vi "StorageRefnumProbe.vi"(1 "dup storage refnum":refnum<k20>) -> (0 "stop":bool)   [LabVIEW 2017]
uses:
  <resource>/objmgr/Storage.rc
panel:
  in  "Invalid refnum":string="INVALID REFNUM"
  in  "Tab Control":T1(tab)
  in  "Storage parameters":i32(listbox)
  out "USI Storage type":string
  out "Object type:":string
  in  "Properties":i32(listbox)
  in  "Data values":i32(listbox)
  out "Waveform Graph":dynamicdata(graph)
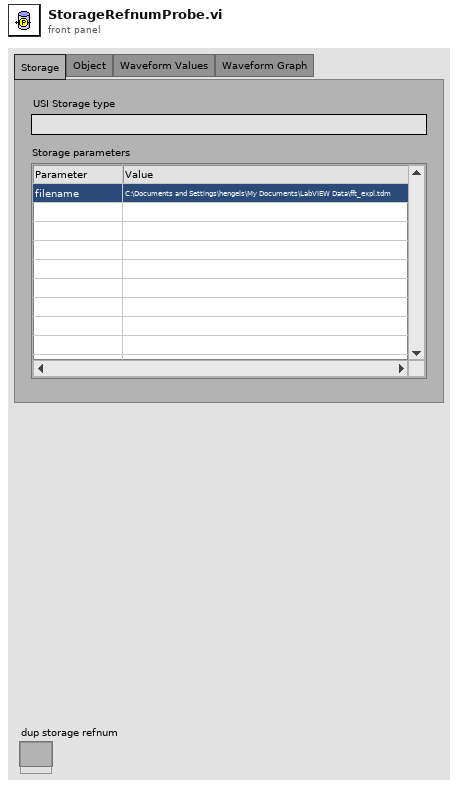
[diagram p1: front panel]
types:
  T1 = enum32{"Storage", "Object", "Waveform Values", "Waveform Graph"}
  T2 = enum32{"Page Enabled", "Page Disabled", "Page Disabled & Grayed"}
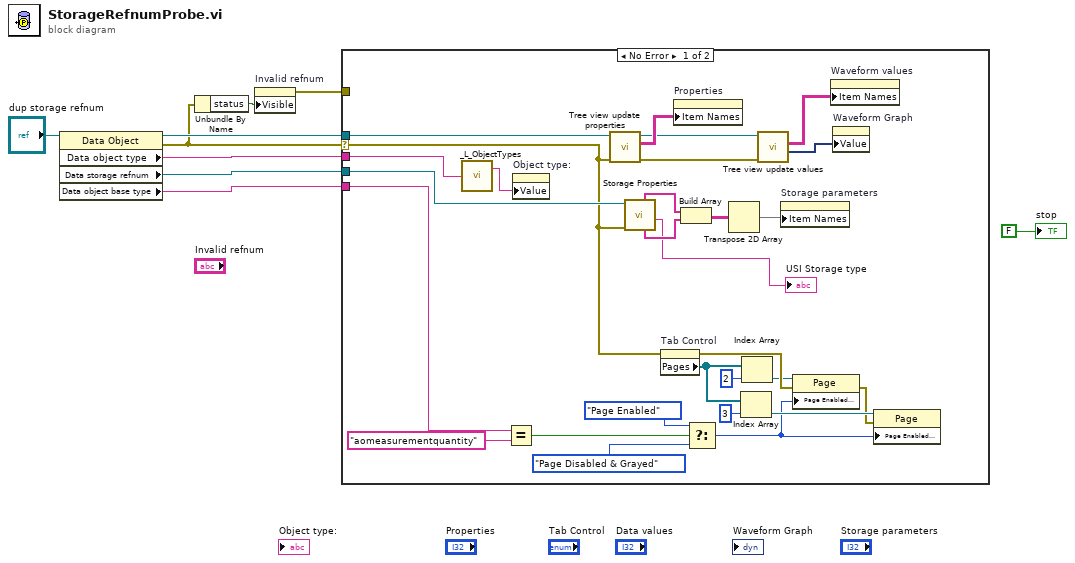
[diagram p0: block diagram]
diagram:
  n1 = property class="Data Object"(reference="dup storage refnum") -> (reference out=w9:refnum<k20>, error out=w3:errorcluster, "Data object type"=w5:string, "Data storage refnum"=w8:refnum<k20>, "Data object base type"=w7:string)  [unwired: 1 in]
  n2 = Unbundle By Name(w3) -> ("status"=w1:bool)
  n3 = property on="Invalid refnum" class="Str"("Visible"=w1) -> (error out=w2:errorcluster)  [unwired: 2 in, 1 out]
  n4 = case shown="No Error" w3 {
    selector: w3 -> [w10 _]
    tunnel: w9 -> [w36 _]
    tunnel: w8 -> [w31 _]
    tunnel: w7 -> [w19 _]
    tunnel: w5 -> [w12 _]
    tunnel: w2 -> [_ _]
    frame No Error {
      n5 = call <vilib>:"_L_ObjectTypes.vi"("DNL_ObjectType"=w12) -> ("DNL_ObjectTypeMapped"=w11:string)  [unwired: 1 out]
      n6 = Equal?(x=w19, y="aomeasurementquantity") -> (x = y?=w17:bool)
      n7 = property on="Object type:" class="Str"("Value"=w11) -> ()  [unwired: 2 in, 2 out]
      n8 = call <vilib>:"Tree view update properties.vi"("error in (no error)"=w10, "Data Object in"=w36) -> ("error out"=w32:errorcluster, "ItemNames"=w37:string[][], "Data Object out"=w33:refnum<k20>)  [unwired: 3 in]
      n9 = call <vilib>:"Storage Properties.vi"("error in (no error)"=w10, "Data storage in"=w31) -> ("Storage type (long)"=→"USI Storage type":string, "Parameter values"=w30:string[], "Parameter names"=w29:string[])  [unwired: 4 in, 3 out]
      n10 = property on="Tab Control" class="TabCtl (strict)"(error in=w10) -> (error out=w26:errorcluster, "Pages"=w22:refnum<vi>[])  [unwired: 1 in, 1 out]
      n11 = property on="Properties" class="MCListbox (strict)"("Item Names"=w37) -> ()  [unwired: 2 in, 2 out]
      n12 = Build Array(w29, w30) -> (w28:string[][])
      n13 = Select(t=T2."Page Enabled" ("Page Enabled State"), s=w17, f=T2."Page Disabled & Grayed" ("Page Enabled State")) -> (s? t:f=w14:T2)
      n14 = Transpose 2D Array(2D array=w28) -> (transposed array=w27:string[][])
      n15 = Index Array(array=w22, index=3) -> (element=w21:refnum<vi>)
      n16 = Index Array(array=w22, index=2) -> (element=w24:refnum<vi>)
      n17 = call <vilib>:"Tree view update values.vi"("error in (no error)"=w32, "Data Object in"=w33) -> ("Dynamic Data"=w34:dynamicdata, "Values as String array"=w35:string[][])  [unwired: 2 in, 2 out]
      n18 = property on="Storage parameters" class="MCListbox (strict)"("Item Names"=w27) -> ()  [unwired: 2 in, 2 out]
      n19 = property class="Page"(reference=w24, error in=w26, "Page Enabled State"=w14) -> (error out=w20:errorcluster)  [unwired: 1 out]
      n20 = property on="Waveform values" class="MCListbox (strict)"("Item Names"=w35) -> ()  [unwired: 2 in, 2 out]
      n21 = property on="Waveform Graph" class="WFGraph (strict)"("Value"=w34) -> ()  [unwired: 2 in, 2 out]
      n22 = property class="Page"(reference=w21, error in=w20, "Page Enabled State"=w14) -> ()  [unwired: 2 out]
    }
    frame Error {
    }
  }
  "stop" <- FALSE
